vi "Read IsOpen.vi"(8 "error in (no error)":errorcluster, 11 "PIDController in":refnum<class "PIDController.lvclass">) -> (0 "error out":errorcluster, 2 "IsOpen":bool, 3 "PIDController out":refnum<class "PIDController.lvclass">)   [LabVIEW 2023, in "PIDController.lvclass"]
uses:
  PIDController.lvclass
  PIDController.lvclass/PIDController.ctl
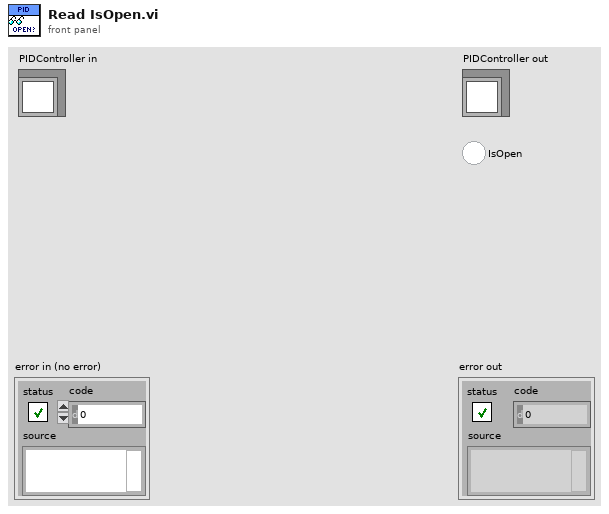
[diagram p1: front panel]
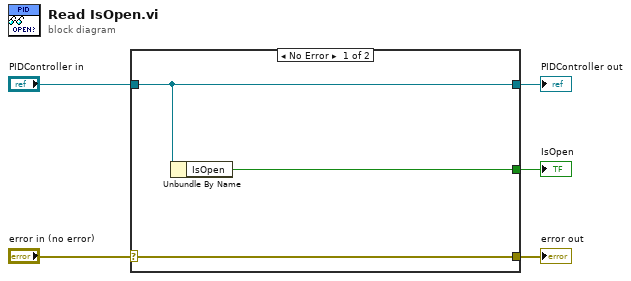
[diagram p0: block diagram]
diagram:
  n1 = case shown="No Error" "error in (no error)" {
    selector: "error in (no error)" -> [w8 w9]
    tunnel: [w8 w9] -> w4
    tunnel: [w7 w10] -> w2
    tunnel: "PIDController in" -> [w7 w10]
    tunnel: [w6 _] -> w1
    frame No Error {
      n2 = Unbundle By Name(w7) -> ("IsOpen"=w6:bool)
    }
    frame Error {
    }
  }
  "error out" <- w4
  "PIDController out" <- w2
  "IsOpen" <- w1
